vi "GetTestItems.vi"(8 "error in":errorcluster caption="错误输入（无错误）", 11 "产品型号":refnum<vi>) -> (0 "error out":errorcluster, 4 "data":string[](array[string]))   [LabVIEW 2013]
uses:
  <vilib>/Utility/NIReport.llb/NI_report.lvclass
  GlobValue.vi
  <vilib>/addons/_office/excel.llb/Excel Get Data ([str]).vi
  <vilib>/addons/_office/NI_ReportGenerationToolkit.lvlib
  <vilib>/Utility/NIReport.llb/Excel/NI_Excel.lvclass
panel:
  out "测试项目":string[][](array[string])
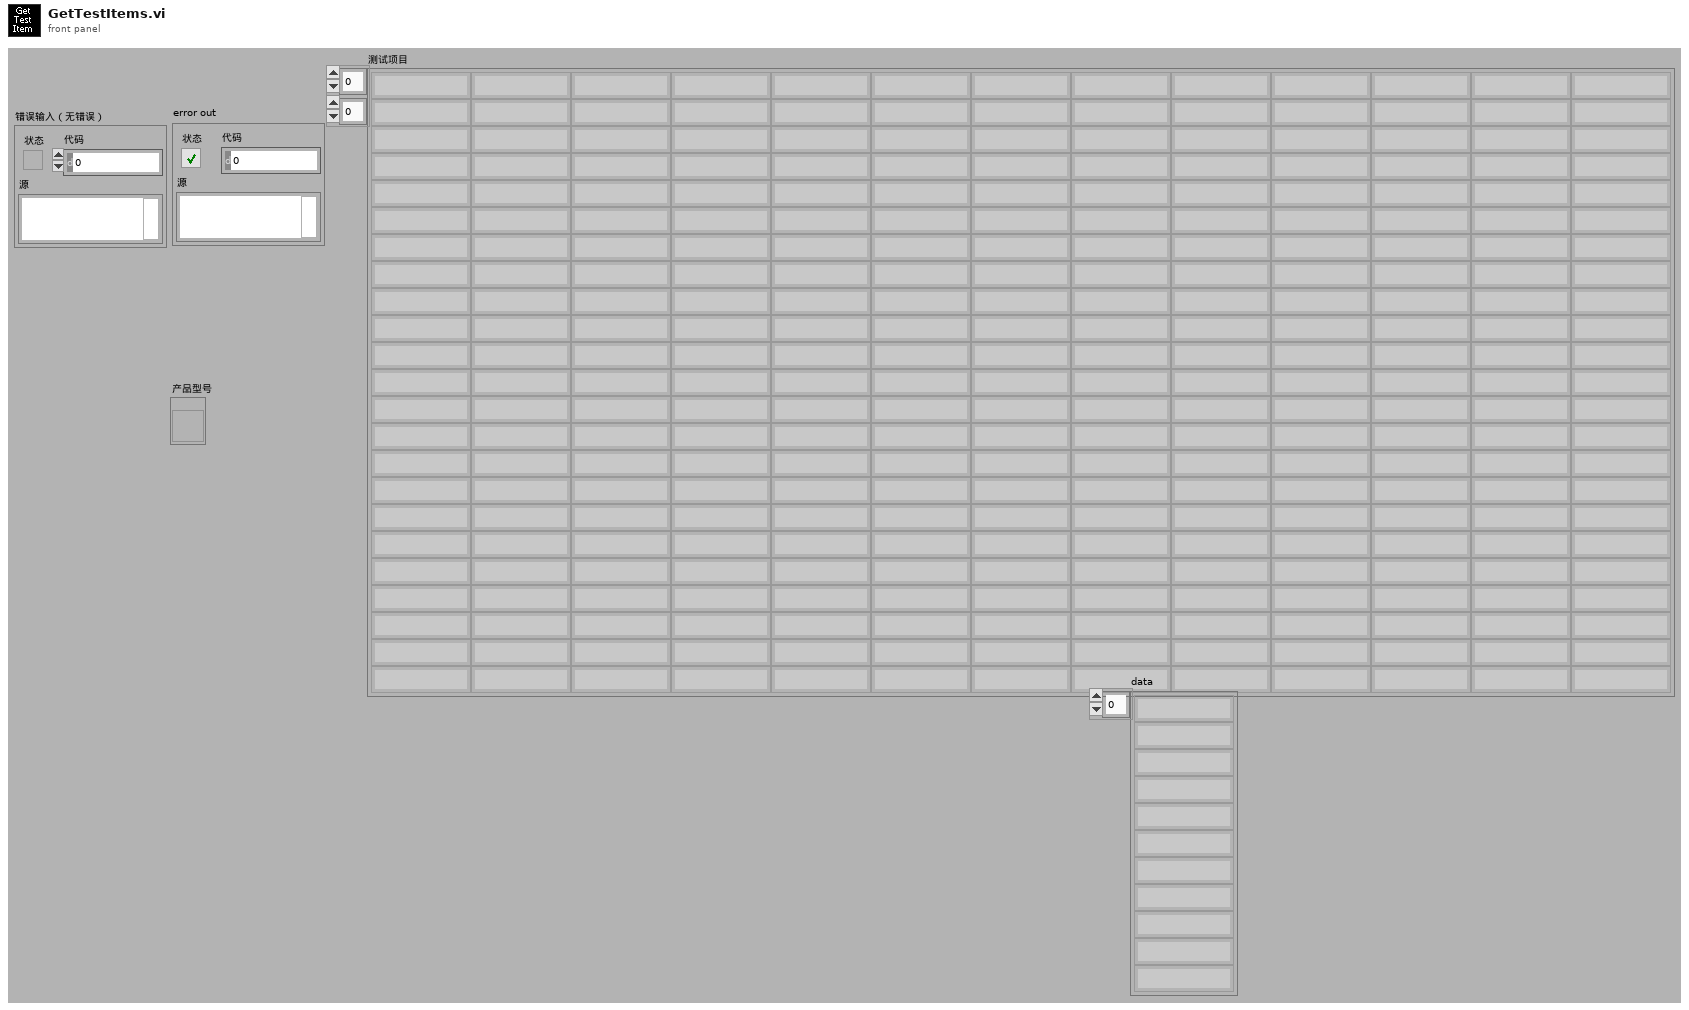
[diagram p1: front panel]
types:
  T1 = enum16{"maximized", "minimized", "normal", "no change"}
  T2 = enum16{"Standard Report", "HTML", "Word", "Excel"}
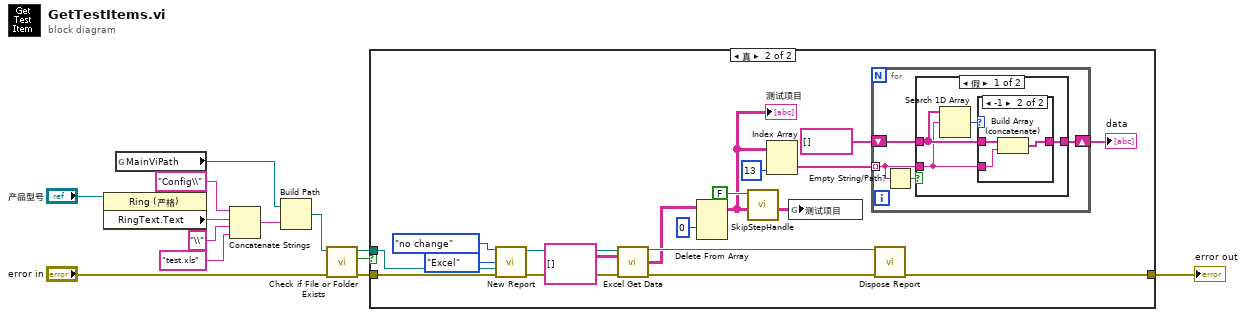
[diagram p0: block diagram]
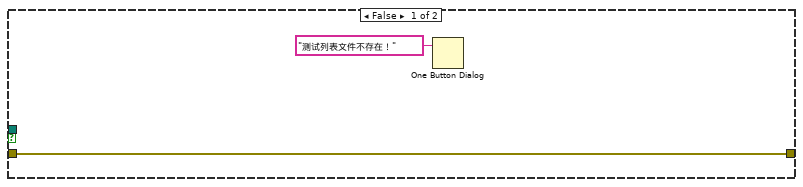
[diagram p2: hidden frame]
diagram:
  n1 = property on="属性节点" class="Ring (严格)"(reference="产品型号") -> ("RingText.Text"=w4:string)  [unwired: 1 in, 2 out]
  n2 = global read "GlobValue.vi" "MainViPath"() -> (w6:path)
  n3 = Concatenate Strings("Config\\" ("字符串"), w4, "\\" ("字符串"), "test.xls" ("字符串")) -> (w2:string)
  n4 = Build Path(base path=w6, name or relative path=w2) -> (appended path=w11:path)
  n5 = call <vilib>:"Check if File or Folder Exists.vi"("error in (no error)"="error in", "path"=w11) -> ("error out"=w10:errorcluster, "file or folder exists?"=w13:bool, "dup path"=w12:path)  [unwired: 7 out]
  n6 = case shown="真" w13 {
    tunnel: w10 -> [w15 w33]
    tunnel: w12 -> [_ w34]
    tunnel: [w15 w31] -> w9
    frame False {
      n7 = One Button Dialog(message="测试列表文件不存在！" ("消息")) -> ()  [unwired: 1 in, 1 out]
    }
    frame True {
      n8 = call <vilib>:"New Report.vi"("window state (normal)"=T1."no change", "report type"=T2."Excel", "template (empty)"=w34, "error in (no error)"=w33) -> ("report out"=w28:refnum<class "NI_report.lvclass">, "error out"=w27:errorcluster)  [unwired: 2 in, 8 out]
      n9 = call-poly <vilib>:"Excel Get Data.vi"("report in"=w28, "data type"=string[][] [], "error in (no error)"=w27) -> ("report out"=w32:refnum<class "NI_report.lvclass">, "data"=w26:string[][], "error out"=w23:errorcluster)  [unwired: 10 in]
      n10 = Delete From Array(array=w26, index (row)=0 ("索引 (行)")) -> (array with subset deleted=w20:string[][])  [unwired: 2 in, 1 out]
      "测试项目" <- w20
      n11 = call "SkipStepHandle.vi"("ItemNamesIn"=w20, "ShowSkipStep?"=FALSE) -> ("ItemNamesOut"=w21:string[][])  [unwired: 9 in]
      n12 = Index Array(array=w20, index (col)=13 ("禁用的索引 (列)")) -> (element=w16:string[])  [unwired: 1 in]
      n13 = global write "GlobValue.vi" "测试项目"(w21) -> ()
      n14 = for "For循环" {
        shift-right: [w37] -> w17
        shift-left: string[] [] -> [w38]
        tunnel: w16 -> [w36] mode=indexing
        n15 = Empty String/Path?(string/path=w36) -> (empty?=w35:bool)
        n16 = case shown="假" w35 {
          tunnel: w38 -> [w41 w47]
          tunnel: [w40 w47] -> w37
          tunnel: w36 -> [w39 _]
          frame False {
            n17 = Search 1D Array(1D array=w41, element=w39) -> (index of element=w42:i32)  [unwired: 1 in]
            n18 = case shown="-1" w42 {
              tunnel: w41 -> [w43 w45]
              tunnel: [w43 w44] -> w40
              tunnel: w39 -> [_ w46]
              frame 1, Default {
              }
              frame -1 {
                n19 = Build Array (concatenate)(w45, w46) -> (w44:string[])
              }
            }
          }
          frame True {
          }
        }
      }
      "data" <- w17
      n20 = call-dynamic "Dispose Report.vi"("report in"=w32, "error in (no error)"=w23) -> ("error out"=w31:errorcluster)  [unwired: 3 in, 10 out]
    }
  }
  "error out" <- w9
